vi "ReadAll.vi"(8 "error in (no error)":errorcluster, 11 "aparCfg in":refnum<class "aparCfg.lvclass">) -> (0 "error out":errorcluster, 1 "ACConfig":T3={"Board 1 alias"="192.168.1.110", "Board 1 Enable"=FALSE, "Board 2 alias"="192.168.1.110", "Board 2 Enable"=FALSE}, 2 "N5222A Cfg":T4={"ResourceName"="", "Enable"=FALSE, "Channel"=1, "CalFileName"="", "MeasName"="", "TempDatFile"="", "Power, dBm"=-30.0, "NumPoints"=201, "Start Freq, Hz"=5000000000.0, "Stop Freq, Hz"=6000000000.0, "NumAverages"=20, "Sweep Type"=0} {"Sweep Type" items=["Linear Frequency", "Log Frequency", "Power Sweep", "CW Time"]; "Stop Freq, Hz" format="%_3p"; "Start Freq, Hz" format="%_3p"}, 3 "aparCfg out":refnum<class "aparCfg.lvclass">, 4 "SequenceConfig":T1, 5 "DataLogConfig":T2)   [LabVIEW 2018, in "aparCfg.lvclass"]
uses:
  aparCfg.lvclass
  N5222A PNA/N5222AConfig.ctl
  ArrayController/ACConfig.ctl
  Datalog/DataLogConfig.ctl
  Sequence/seqConfig.ctl
  aparCfg.lvclass/aparCfg.ctl
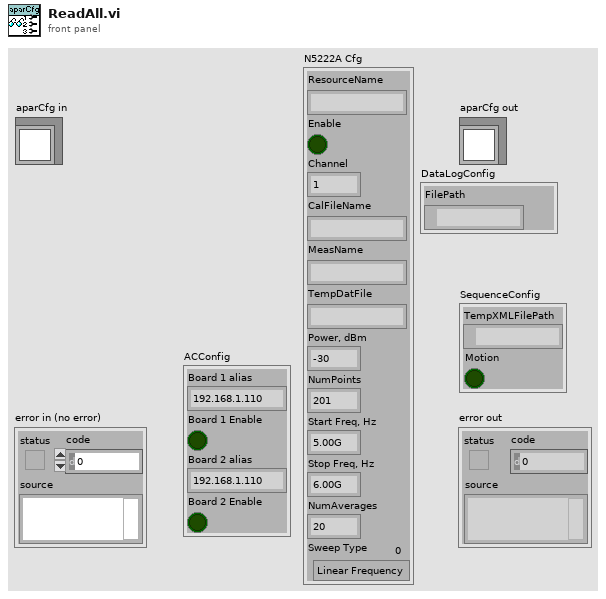
[diagram p1: front panel]
types:
  T1 = typedef "seqConfig.ctl" = cluster{"TempXMLFilePath":path, "Motion":bool}
  T2 = typedef "DataLogConfig.ctl" = cluster{"FilePath":path}
  T3 = typedef "ACConfig.ctl" = cluster{"Board 1 alias":string, "Board 1 Enable":bool, "Board 2 alias":string, "Board 2 Enable":bool}
  T4 = typedef "N5222AConfig.ctl" = cluster{"ResourceName":string, "Enable":bool, "Channel":i32, "CalFileName":string, "MeasName":string, "TempDatFile":string, "Power, dBm":dbl, "NumPoints":i32, "Start Freq, Hz":dbl, "Stop Freq, Hz":dbl, "NumAverages":i32, "Sweep Type":i32}
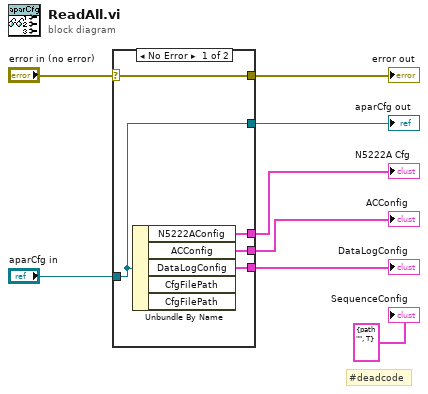
[diagram p0: block diagram]
diagram:
  # "#deadcode"
  n1 = case shown="No Error" "error in (no error)" {
    selector: "error in (no error)" -> [w13 w15]
    tunnel: [w13 w15] -> w7
    tunnel: [w12 w14] -> w5
    tunnel: "aparCfg in" -> [w12 w14]
    tunnel: [w11 _] -> w4
    tunnel: [w10 _] -> w3
    tunnel: [w9 _] -> w2
    frame No Error {
      n2 = Unbundle By Name(w12) -> ("N5222AConfig"=w11:T4, "ACConfig"=w10:T3, "DataLogConfig"=w9:T2)  [unwired: 2 out]
    }
    frame Error {
    }
  }
  "error out" <- w7
  "aparCfg out" <- w5
  "N5222A Cfg" <- w4
  "ACConfig" <- w3
  "DataLogConfig" <- w2
  "SequenceConfig" <- T1 {"TempXMLFilePath"=path "", "Motion"=TRUE} ("SequenceConfig")
